vi "CB Flywheel Model.vi"(5 "J (moment of intertia)":dbl, 6 "encoder?":bool=TRUE, 7 "G (gear ratio)":dbl, 8 "dt":dbl=-1.0, 10 "num motors":i32=1, 11 "Motor ID":T3) -> (3 "Discrete SSM":T1)   [LabVIEW 2020]
uses:
  Motors/CB Motor ID.ctl
  CB State Space.ctl
  <vilib>/Analysis/Matrix/Datatypes/RealMatrix.ctl
  <vilib>/Analysis/Matrix/NI_Matrix.lvlib
panel:
  out "State Space Model":T1
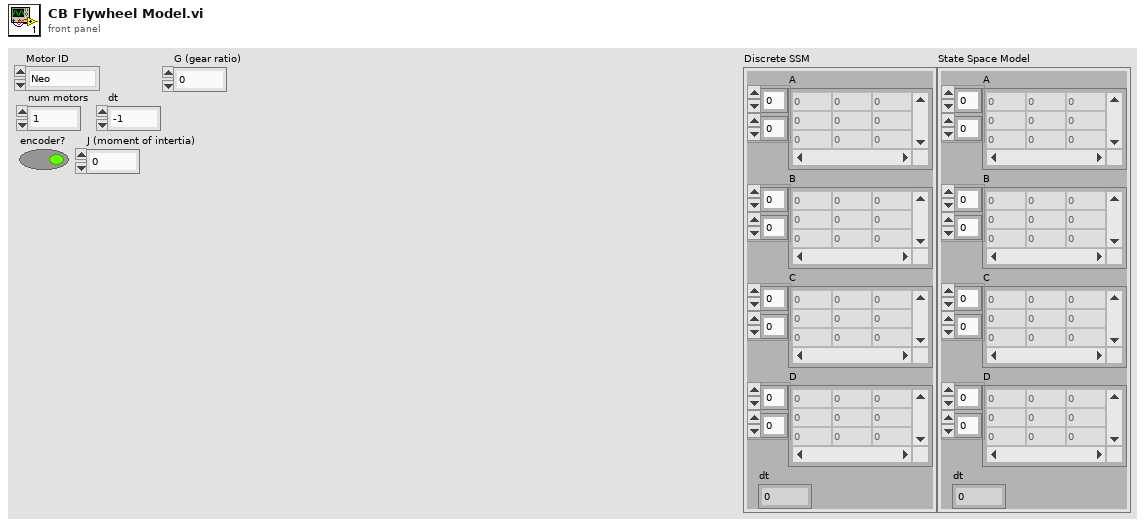
[diagram p1: front panel]
types:
  T1 = typedef "CB State Space.ctl" = cluster{"A":T2, "B":T2, "C":T2, "D":T2, "dt":dbl}
  T2 = typedef "NI_Matrix.lvlib/RealMatrix.ctl" = dbl[][]
  T3 = typedef "CB Motor ID.ctl" = enum16{"Neo", "Neo 550", "Falcon 500", "775pro"}
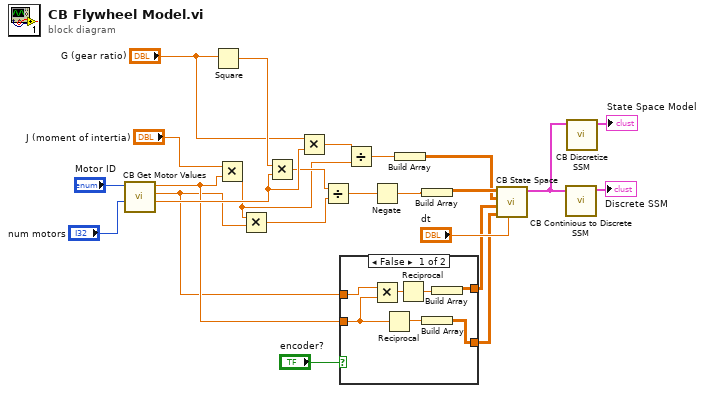
[diagram p0: block diagram]
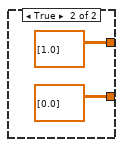
[diagram p2: hidden frame]
diagram:
  n1 = call "CB Get Motor Values.vi"("num motors"="num motors", "Motor ID"="Motor ID") -> ("Kt"=w16:dbl, "Kv"=w6:dbl, "R"=w7:dbl)  [unwired: 6 in, 1 out]
  n2 = Square(x="G (gear ratio)") -> (x^2=w17:dbl)
  n3 = Multiply(x="J (moment of intertia)", y=w7) -> (x*y=w10:dbl)
  n4 = Multiply(x=w10, y=w6) -> (x*y=w12:dbl)
  n5 = Multiply(x=w17, y=w16) -> (x*y=w13:dbl)
  n6 = Multiply(x="G (gear ratio)", y=w16) -> (x*y=w11:dbl)
  n7 = Divide(x=w13, y=w12) -> (x/y=w4:dbl)
  n8 = case shown="False" "encoder?" {
    tunnel: [w25 T2 [[1.0]] ("C")] -> w20
    tunnel: [w30 T2 [[0.0]] ("D")] -> w19
    tunnel: w7 -> [w29 _]
    tunnel: w6 -> [w28 _]
    frame False {
      n9 = Multiply(x=w28, y=w29) -> (x*y=w27:dbl)
      n10 = Reciprocal(x=w29) -> (1/x=w31:dbl)
      n11 = Reciprocal(x=w27) -> (1/x=w26:dbl)
      n12 = Build Array(w31) -> (w30:T2)
      n13 = Build Array(w26) -> (w25:T2)
    }
    frame True {
    }
  }
  n14 = Divide(x=w11, y=w10) -> (x/y=w5:dbl)
  n15 = Negate(x=w4) -> (-x=w3:dbl)
  n16 = Build Array(w5) -> (w8:T2)
  n17 = Build Array(w3) -> (w9:T2)
  n18 = call "CB State Space.vi"("dt"="dt", "D"=w19, "C"=w20, "B"=w8, "A"=w9) -> ("State Space Model"=w2:T1)  [unwired: 5 in, 1 out]
  n19 = call "CB Continious to Discrete SSM.vi"("Cont SSM"=w2) -> ("Discrete SSM"=→"Discrete SSM":T1)  [unwired: 10 in]
  n20 = call "CB Discretize SSM.vi"("Cont SSM"=w2) -> ("State Space Model"=→"State Space Model":T1)  [unwired: 10 in]
